vi "main.vi"() -> ()   [LabVIEW 2023]
doc: "VI sluzy do wyznaczania odpowiedzi filtru IIR. Program sklada sie z subvi sluzacego do generowania sygnalu oraz subvi generujace odpowiedz filtru. \n\nDo wyboru przez uzytkownika jest typ sygnalu wejsciowego: sinusoidalny, prostokatny, trójkatny oraz pilooidalny. Uzytkownik powininen równiez wybrac dewiacje sygnalu Gaussa, który symuluje zaklocenia sygnalu wejsciowego, czestotliwosc, opoznienie oraz amplitude.\n\nZatrzymanie programu odbywa sie poprzez uzycie przycisku stop. Do prawidlowego dzialania programu wymagane jest zdefiniowanie niezerowych czestotliwosci i amplitudy sygnalu."
uses:
  <vilib>/ptbypt/NI_PtbyPt.lvlib
panel:
  in  "stop":bool
  in  "millisecond multiple":u32
  in  "type_of_signal":T1(ring)
  out "Wykres sygnalu wejsciowego oraz odpowiedzi filtru IIR":cluster{dbl, dbl}(graph)
  in  "standard deviation":dbl=1.0 format="%0.2f"
  in  "Frequency":dbl
  in  "Amplitude":dbl
  in  "Offset":dbl
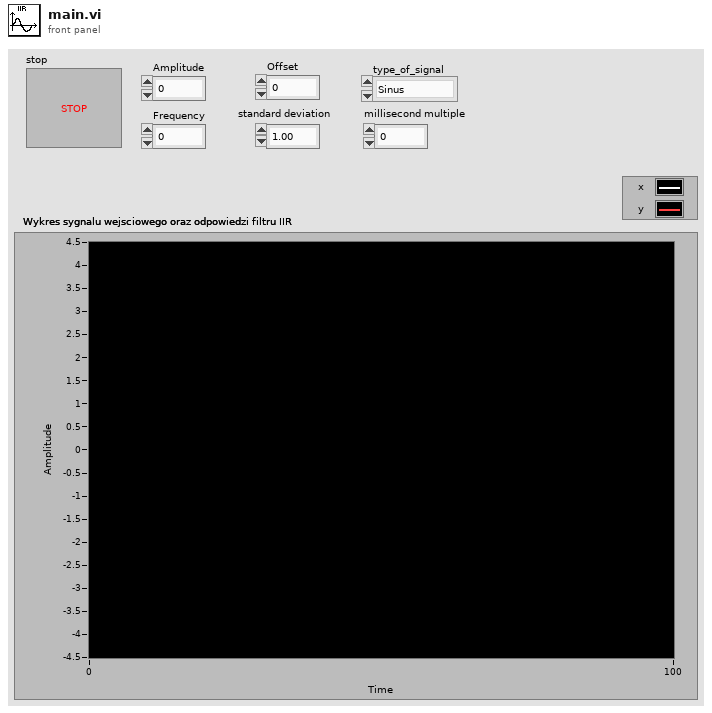
[diagram p1: front panel]
types:
  T1 = enum16{"Sinus", "Rectangle", "Triangle", "Sawthooth"}
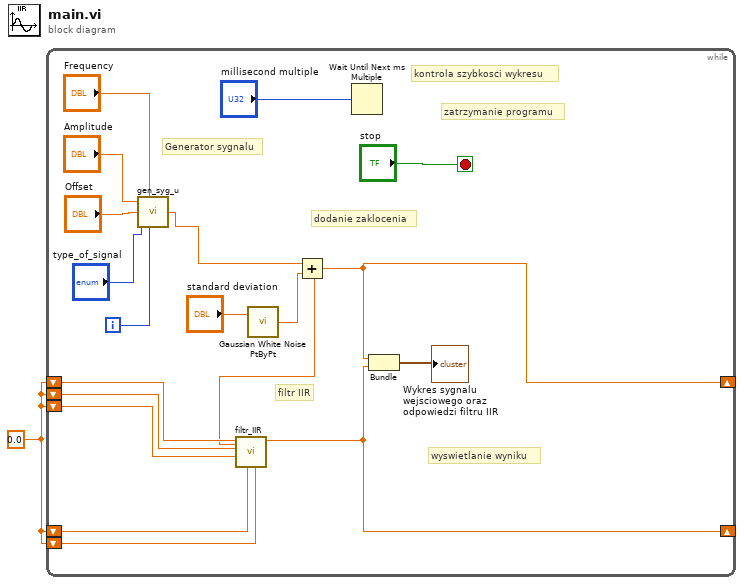
[diagram p0: block diagram]
diagram:
  w1 = 0.0
  n1 = while {
    shift-right: [w11] -> _
    shift-left: w1 -> [w15]
    shift-left: w1 -> [w16]
    shift-left: w1 -> [w17]
    shift-right: [w12] -> _
    shift-left: w1 -> [w13]
    shift-left: w1 -> [w14]
    i -> [w3]
    stop <- "stop" stop-if-true
    # "zatrzymanie programu"
    # "kontrola szybkosci wykresu"
    # "filtr IIR"
    # "wyswietlanie wyniku"
    # "dodanie zaklocenia"
    # "Generator sygnalu"
    n2 = call "gen_syg_u.vi"("Amplituda"="Amplitude", "czestotliwosc"="Frequency", "Offset"="Offset", "rodzaj"="type_of_signal", "probka"=w3) -> ("Wyjscie"=w5:dbl)
    n3 = call <vilib>:"Gaussian White Noise PtByPt.vi"("standard deviation"="standard deviation") -> ("Gaussian white noise"=w18:dbl)  [unwired: 2 in]
    n4 = Add(x=w5, y=w18) -> (x+y=w11:dbl)
    n5 = call "filtr_IIR.vi"("Y_n-2"=w14, "Y_n-1"=w13, "X_n"=w11, "X_n-3"=w17, "X_n-2"=w16, "X_n-1"=w15) -> ("Y_n"=w12:dbl)  [unwired: 5 in]
    n6 = Wait Until Next ms Multiple(millisecond multiple="millisecond multiple") -> ()  [unwired: 1 out]
    n7 = Bundle(w11, "Y_n"=w12) -> (→"Wykres sygnalu wejsciowego oraz odpowiedzi filtru IIR":cluster{dbl, "Y_n":dbl})  [unwired: 1 in]
  }
